vi "sub_数组奇数行转置.vi"(1 "Pulse Number":enum16{"SP", "DP"}(ring)=enum."DP", 2 "Input":u16[][](array[numeric])) -> (0 "output":u16[][](array[numeric]))   [LabVIEW 2015]
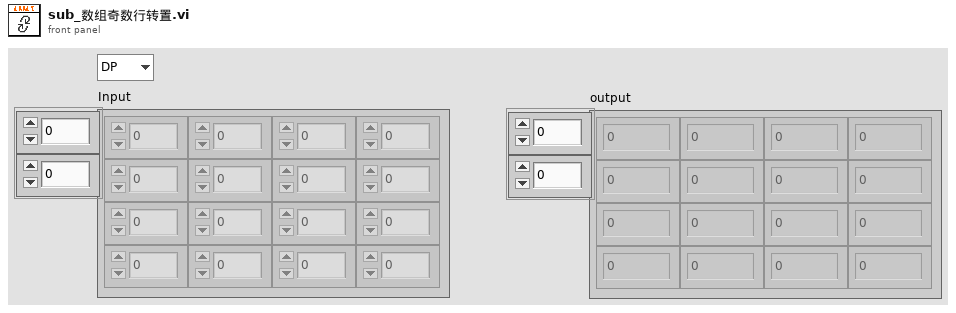
[diagram p1: front panel]
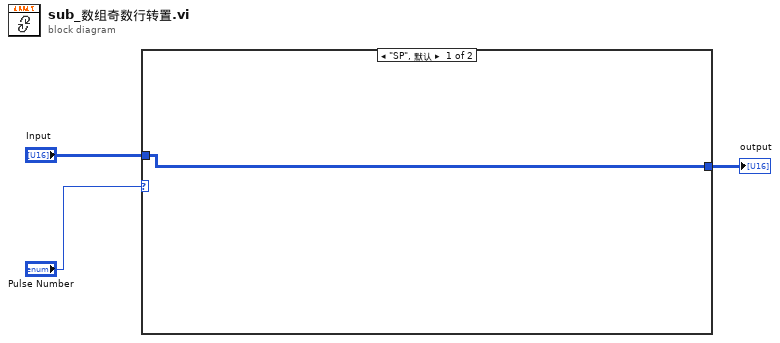
[diagram p0: block diagram]
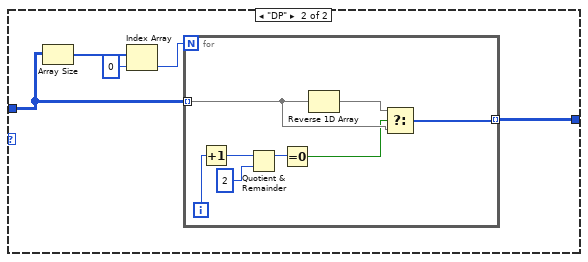
[diagram p2: hidden frame]
diagram:
  n1 = case shown="\"SP\", 默认" "Pulse Number" {
    tunnel: "Input" -> [w4 w6]
    tunnel: [w4 w5] -> w2
    frame "SP", Default {
    }
    frame "DP" {
      n2 = Array Size(array=w6) -> (size(s)=w8:i32[])
      n3 = Index Array(array=w8, index=0 ("索引")) -> (element=w7:i32)
      n4 = for {
        N: w7 -> [_]
        tunnel: w6 -> [w13] mode=indexing
        tunnel: [w11] -> w5 mode=indexing
        i -> [w17]
        n5 = Increment(x=w17) -> (x+1=w10:i32)
        n6 = Quotient & Remainder(x=w10, y=2) -> (x-y*floor(x/y)=w15:i32)  [unwired: 1 out]
        n7 = Equal To 0?(x=w15) -> (x = 0?=w12:bool)
        n8 = Reverse 1D Array(array=w13) -> (reversed array=w14:u16[])
        n9 = Select(t=w14, s=w12, f=w13) -> (s? t:f=w11:u16[])
      }
    }
  }
  "output" <- w2
